vi "Priority.vi"(8 "error in (no error)":errorcluster, 11 "TestQueryAuth in":refnum<class "TestQueryAuth.lvclass">) -> (0 "error out":errorcluster, 2 "Priority":u16, 3 "TestQueryAuth out":refnum<class "TestQueryAuth.lvclass">)   [LabVIEW 2020]
uses:
  TestQueryAuth.lvclass
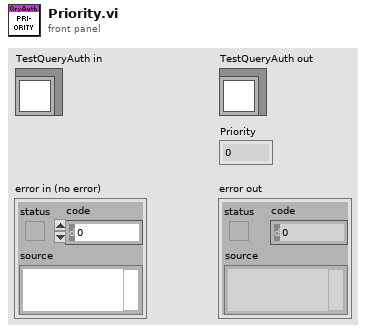
[diagram p1: front panel]
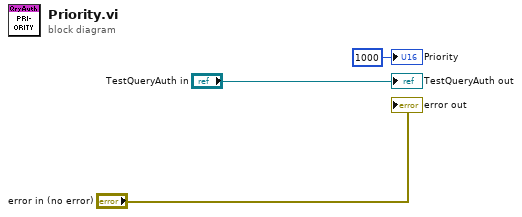
[diagram p0: block diagram]
diagram:
  "error out" <- "error in (no error)"
  "TestQueryAuth out" <- "TestQueryAuth in"
  "Priority" <- u16 1000 ("Priority")
